vi "KGN Get MFC Flows.vi"(8 "Fehler (Eingang, kein Fehler)":errorcluster, 9 "Info Cluster":T1, 10 "VISA-Ressourcenname":refnum<visa-resource-name>, 11 "device (Eingang)":u32) -> (0 "Fehler (Ausgang)":errorcluster, 1 "Info Cluster out":T1, 2 "VISA-Ressourcenname out":refnum<visa-resource-name>, 3 "dup device (Ausgang)":u32, 4 "MFC Flow Cluster":cluster{"min flow":dbl, "max flow":dbl}[](array[cluster]) {"max flow" format="%.2f"; "min flow" format="%.2f"}, 6 "Kommandos gesendet":string)   [LabVIEW 2020, in "Linearisierung v2.lvlib" / "Gasteiler.lvlib" / "HovaCAL_Interface.lvlib" / "KGN.lvlib" / "KGN GUI Get.lvlib"]
uses:
  KGN GUI Get.lvlib
  Controls/Info Cluster.ctl
  get/get.lvlib
  Controls/Controls.lvlib
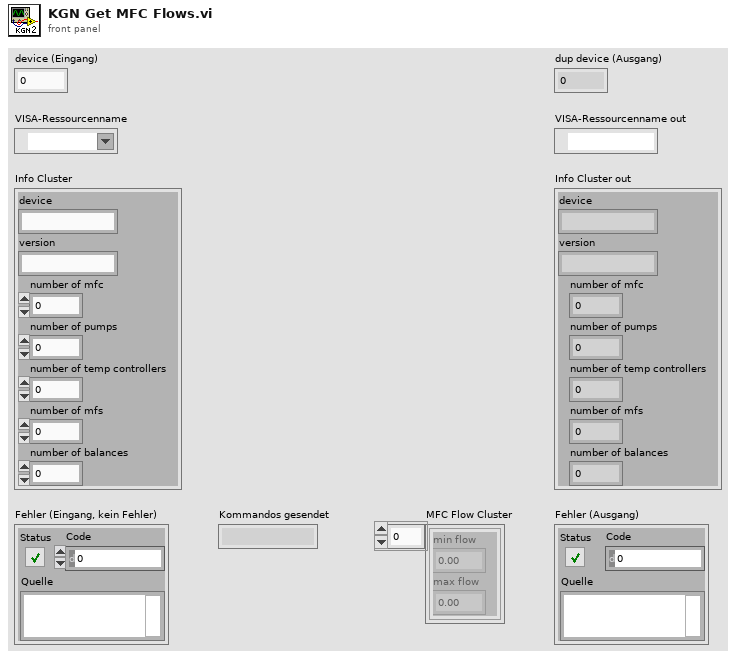
[diagram p1: front panel]
types:
  T1 = typedef "Linearisierung v2.lvlib/Gasteiler.lvlib/HovaCAL_Interface.lvlib/Controls.lvlib/Info Cluster.ctl" = cluster{"device":string, "version":string, "number of mfc":i32, "number of pumps":i32, "number of temp controllers":i32, "number of mfs":i32, "number of balances":i32}
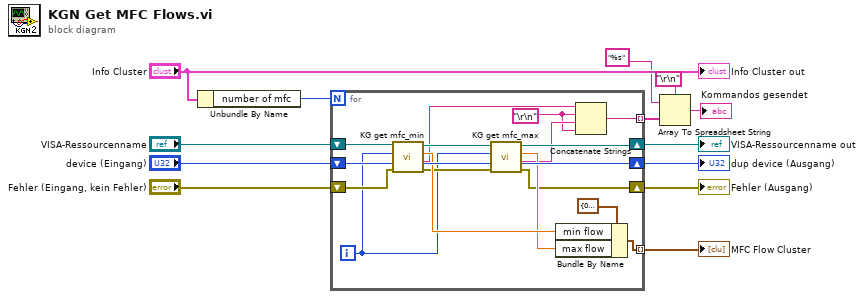
[diagram p0: block diagram]
diagram:
  n1 = Unbundle By Name("Info Cluster") -> ("number of mfc"=w8:i32)
  n2 = for {
    N: w8 -> [_]
    tunnel: [w25] -> w5 mode=indexing
    shift-right: [w19] -> w12
    shift-left: "Fehler (Eingang, kein Fehler)" -> [w29]
    shift-right: [w28] -> w13
    shift-left: "device (Eingang)" -> [w28]
    shift-right: [w21] -> w6
    shift-left: "VISA-Ressourcenname" -> [w24]
    tunnel: [w14] -> w4 mode=indexing
    i -> [w20]
    w15 = "\r\n"
    n3 = call "KG get mfc_min.vi"("Fehler (Eingang, kein Fehler)"=w29, "mfc"=w20, "VISA-Ressourcenname"=w24) -> ("Fehler (Ausgang)"=w23:errorcluster, "Kommando gesendet"=w17:string, "mfc min"=w27:dbl, "VISA-Ressourcenname (Ausgang)"=w22:refnum<visa-resource-name>)  [unwired: 5 in]
    n4 = call "KG get mfc_max.vi"("Fehler (Eingang, kein Fehler)"=w23, "mfc"=w20, "VISA-Ressourcenname"=w22) -> ("Fehler (Ausgang)"=w19:errorcluster, "Kommando gesendet"=w16:string, "mfc max"=w26:dbl, "VISA-Ressourcenname (Ausgang)"=w21:refnum<visa-resource-name>)  [unwired: 5 in]
    n5 = Bundle By Name(cluster=cluster{"min flow":dbl, "max flow":dbl} {"min flow"=0.0, "max flow"=0.0} ("MFC Flow Cluster"), "min flow"=w27, "max flow"=w26) -> (w25:cluster{"min flow":dbl, "max flow":dbl})
    n6 = Concatenate Strings(w17, w15, w16, w15) -> (w14:string)
  }
  "dup device (Ausgang)" <- w13
  "Fehler (Ausgang)" <- w12
  "MFC Flow Cluster" <- w5
  "VISA-Ressourcenname out" <- w6
  n7 = Array To Spreadsheet String(delimiter (Tab)="\r\n", array=w4, 3:"%s" ("Format-String")) -> (spreadsheet string=→"Kommandos gesendet":string)
  "Info Cluster out" <- "Info Cluster"
